vi "CamControl.vi"() -> ()   [LabVIEW 2016]
uses:
  <vilib>/userdefined/High Color/IMAQdx.ctl
  <vilib>/vision/driver/NI_Vision_Acquisition_Software.lvlib
  <resource>/objmgr/imaqdx.rc
panel:
  in  "Slide":dbl(slide) scale=0.00024415..0.125
  in  "ValueDBL":dbl=0.00024415 min=0.00024415 max=0.125 step=0.0001
  out "error out 4":errorcluster
  in  "Path":path
  in  "stop":bool
  in  "Boolean":bool
  out "error out 3":errorcluster
  out "Image":T1(plugin-control)
  out "error out 2":errorcluster
  out "error out":errorcluster
  in  "Session In":T2
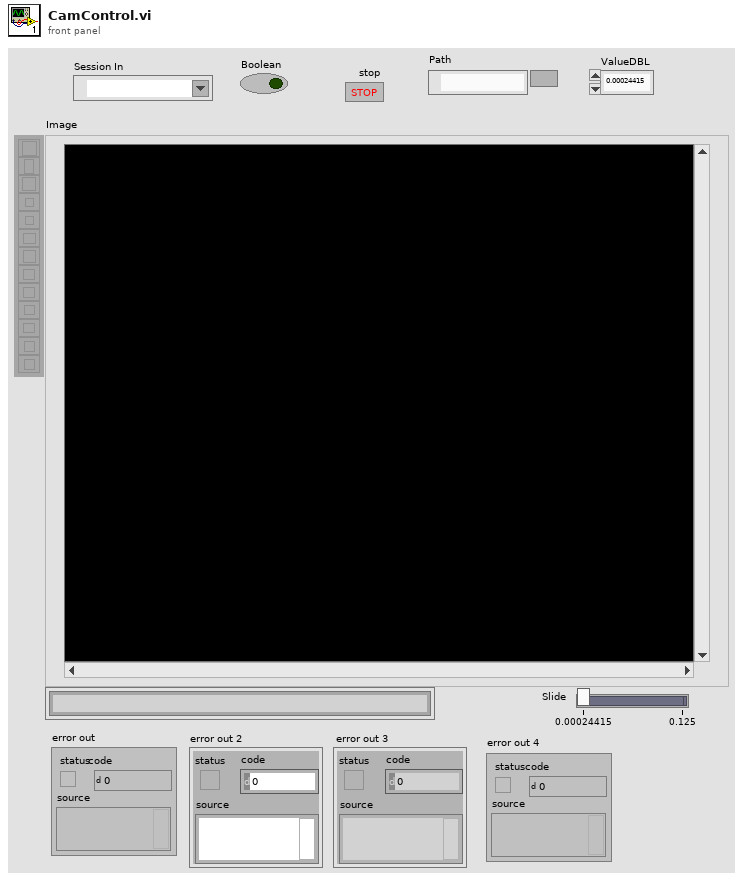
[diagram p1: front panel]
types:
  T1 = typedef "IMAQ Image.ctl" = refnum<image>
  T2 = typedef "IMAQdx.ctl" = refnum<k21>
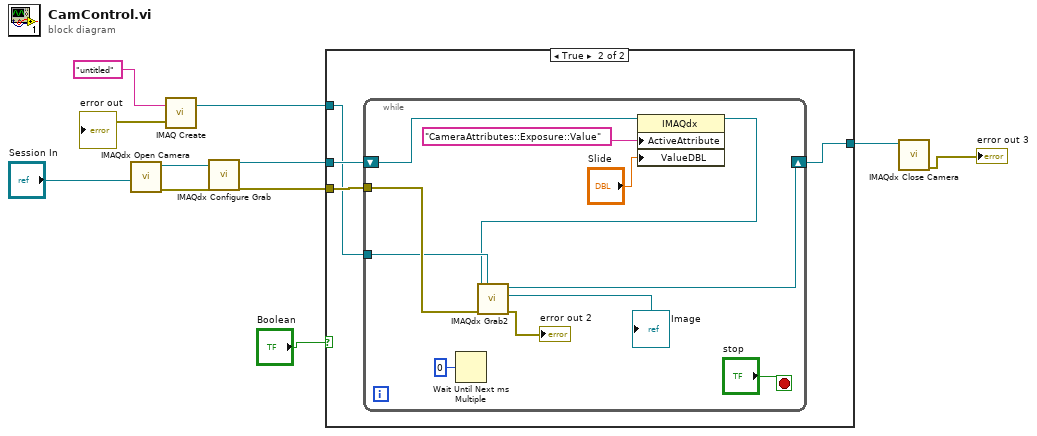
[diagram p0: block diagram]
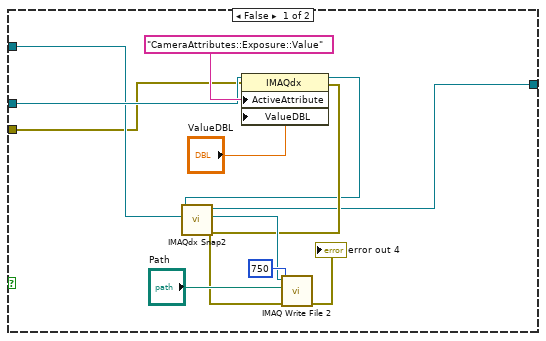
[diagram p2: hidden frame]
diagram:
  n1 = call <vilib>:"IMAQdx Open Camera.vi"("Session In"="Session In") -> ("error out"=w10:errorcluster, "Session Out"=w2:T2)  [unwired: 9 in]
  n2 = call "IMAQ Create"("Image Name"="untitled") -> ("New Image"=w4:T1, "error out"=→"error out":errorcluster)  [unwired: 4 in]
  n3 = call <vilib>:"IMAQdx Configure Grab.vi"("error in"=w10, "Session In"=w2) -> ("error out"=w6:errorcluster, "Session Out"=w9:T2)  [unwired: 8 in]
  n4 = case shown="True" "Boolean" {
    tunnel: w9 -> [w15 w28]
    tunnel: [w12 w25] -> w7
    tunnel: w6 -> [w13 w27]
    tunnel: w4 -> [w14 w26]
    frame False {
      n5 = property class="IMAQdx"(reference=w15, error in=w13, "ActiveAttribute"="CameraAttributes::Exposure::Value", "ValueDBL"="ValueDBL") -> (reference out=w16:T2, error out=w20:errorcluster)
      n6 = call <vilib>:"IMAQdx Snap2.vi"("error in"=w20, "Image In"=w14, "Session In"=w16) -> ("error out"=w19:errorcluster, "Image Out"=w21:T1, "Session Out"=w12:T2)  [unwired: 6 in]
      n7 = call-poly "IMAQ Write File 2"("error in (no error)"=w19, "Image Quality"=u32 750, "File Path"="Path", "Image"=w21) -> ("error out"=→"error out 4":errorcluster)  [unwired: 6 in, 1 out]
    }
    frame True {
      n8 = while {
        tunnel: w27 -> [w39]
        tunnel: w26 -> [w38]
        shift-right: [w34] -> w25
        shift-left: w28 -> [w31]
        stop <- "stop" stop-if-true
        n9 = Wait Until Next ms Multiple(millisecond multiple=u32 0) -> ()  [unwired: 1 out]
        n10 = property class="IMAQdx"(reference=w31, "ActiveAttribute"="CameraAttributes::Exposure::Value", "ValueDBL"="Slide") -> (reference out=w30:T2)  [unwired: 1 in, 1 out]
        n11 = call <vilib>:"IMAQdx Grab2.vi"("error in"=w39, "Image In"=w38, "Session In"=w30) -> ("error out"=→"error out 2":errorcluster, "Image Out"=→"Image":T1, "Session Out"=w34:T2)  [unwired: 5 in, 1 out]
      }
    }
  }
  n12 = call <vilib>:"IMAQdx Close Camera.vi"("Session In"=w7) -> ("error out"=→"error out 3":errorcluster)  [unwired: 10 in]
